vi "程序设置-新建程序.vi"(0 "Program NO.":string) -> (14 "Cancelled?":bool caption="取消？")   [LabVIEW 2017]
doc: "该模板用于创建能够进行事件处理的对话框。"
panel:
  in  "Sequence":bool
  in  "Explanation":string
  in  "Symbol":string
  in  "Index":i32
  out "程序注释 2":string
  out "是否保存":bool
  out "错误输出":errorcluster caption="错误输入"
  in  "程序列表":i32(ring)
  in  "程序注释":string
  in  "Cancel":bool caption="取消"
  in  "Create":bool caption="确定"
  # "新建程序"
  # "程序列表："
  # "程序号  ："
  # "程序注释："
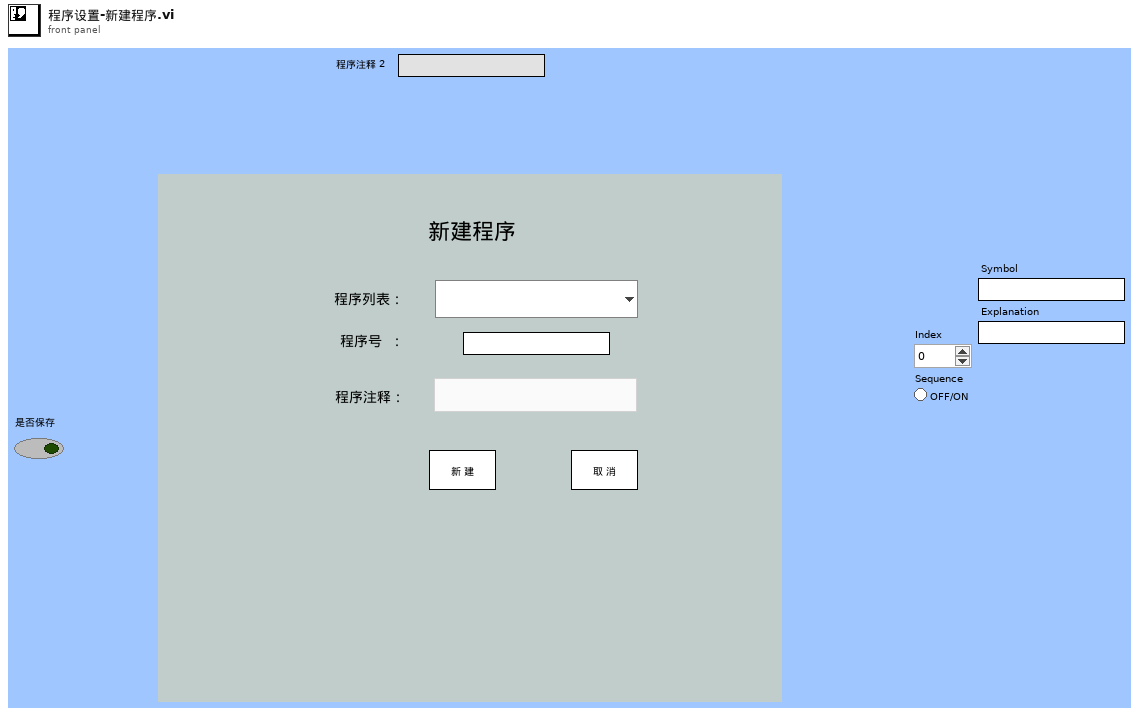
[diagram p1: front panel]
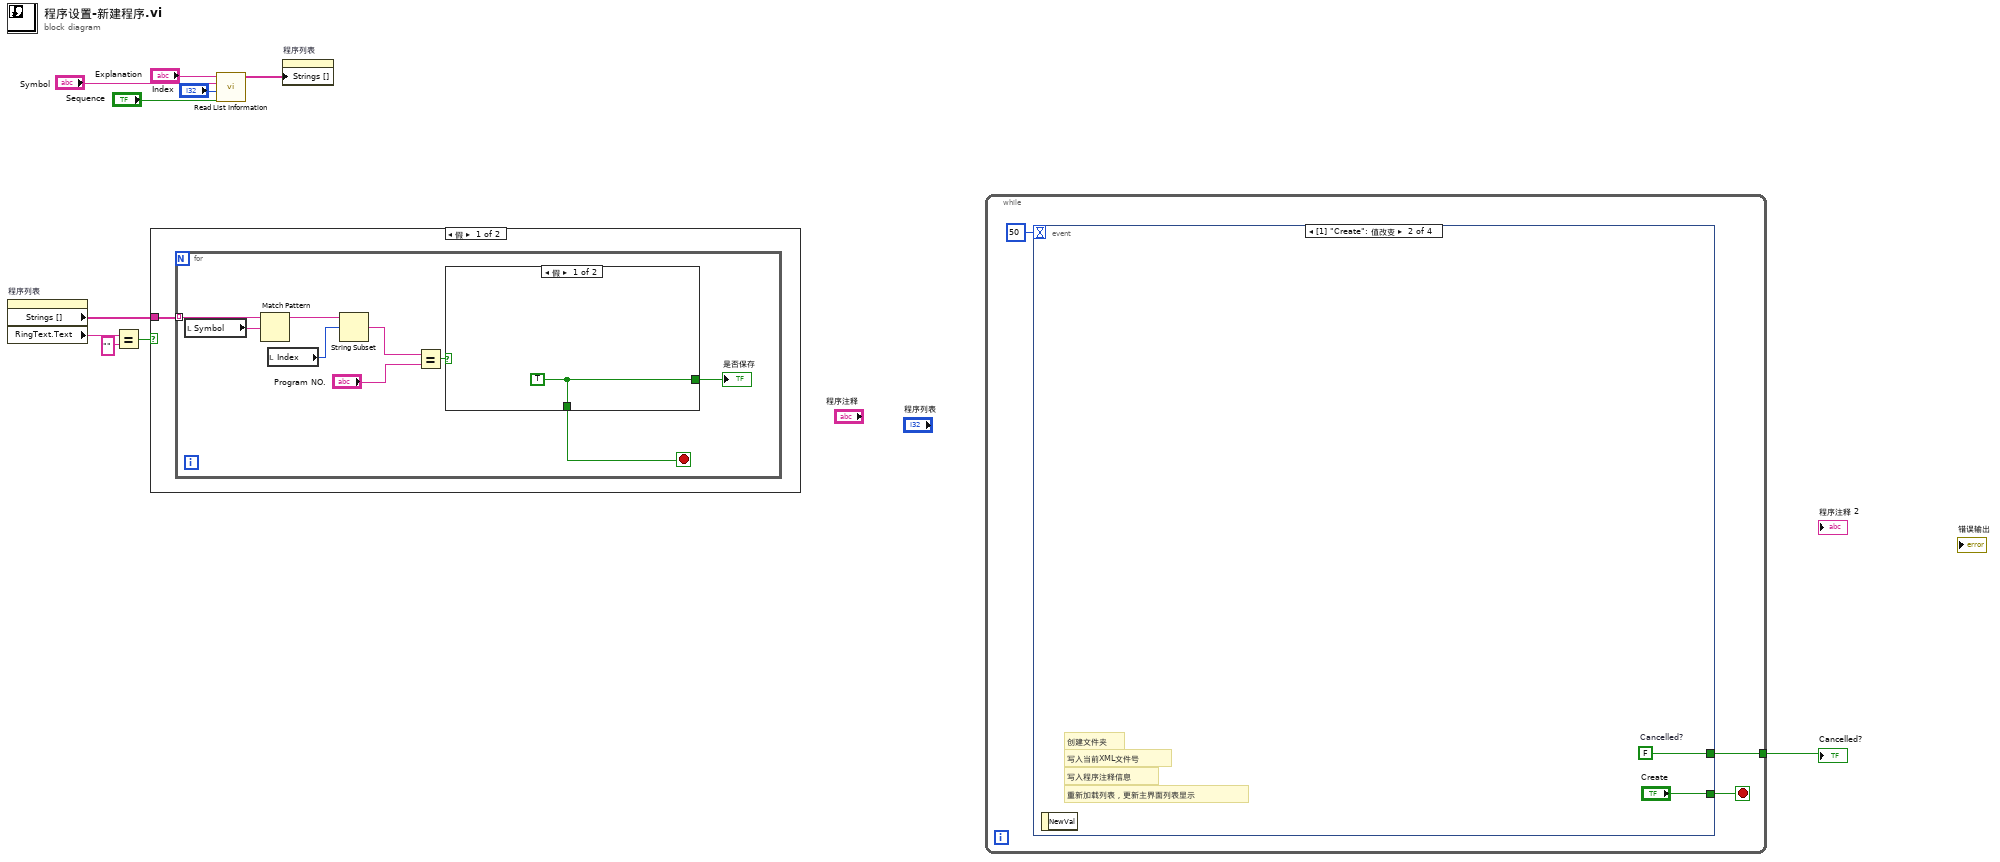
[diagram p0: block diagram]
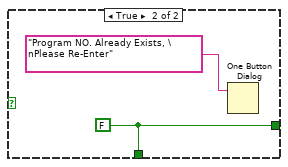
[diagram p2: hidden frame]
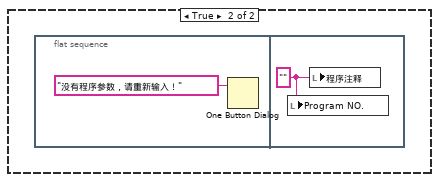
[diagram p3: hidden frame]
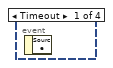
[diagram p4: hidden frame]
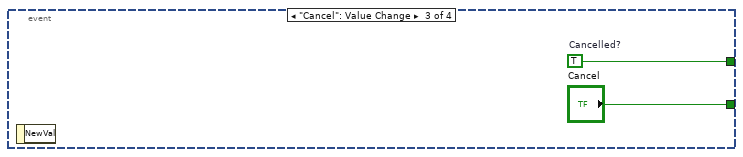
[diagram p5: hidden frame]
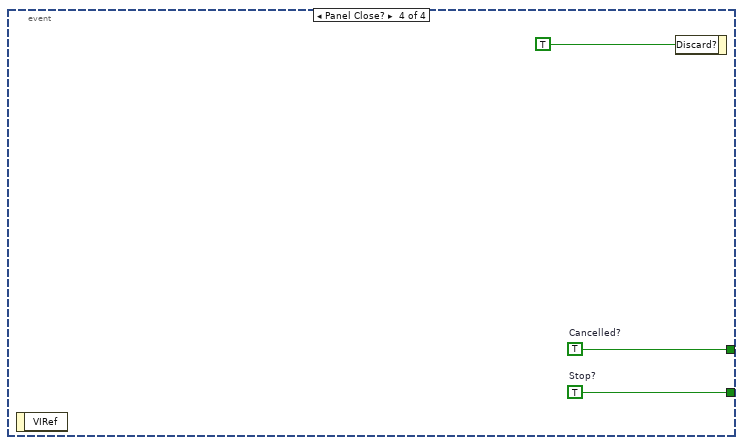
[diagram p6: hidden frame]
diagram:
  n1 = property on="程序列表" class="Ring (严格)"() -> ("Strings []"=w6:string[], "RingText.Text"=w7:string)  [unwired: 2 in, 2 out]
  n2 = Equal?(x=w7, y="") -> (x = y?=w9:bool)
  n3 = case shown="假" w9 {
    tunnel: w6 -> [w11 _]
    frame False {
      n4 = for {
        tunnel: w11 -> [w17] mode=indexing
        stop <- w20 stop-if-true
        n5 = local read "Symbol"() -> (w16:string)
        n6 = Match Pattern(string=w17, regular expression=w16) -> (before substring=w15:string)  [unwired: 1 in, 3 out]
        n7 = local read "Index"() -> (w14:i32)
        n8 = String Subset(string=w15, offset (0)=w14) -> (substring=w13:string)  [unwired: 1 in]
        n9 = Equal?(x=w13, y="Program NO.") -> (x = y?=w18:bool)
        n10 = case shown="假" w18 {
          tunnel: [w21 w23] -> w20
          tunnel: [w21 w23] -> w19
          frame False {
            w21 = TRUE ("程序是否存在")
          }
          frame True {
            w23 = FALSE ("程序是否存在")
            n11 = One Button Dialog(message="Program NO. Already Exists, \nPlease Re-Enter" ("消息")) -> ()  [unwired: 1 in, 1 out]
          }
        }
        "是否保存" <- w19
      }
    }
    frame True {
      n12 = flat-sequence {
        frame #0 {
          n13 = One Button Dialog(message="没有程序参数，请重新输入！" ("消息")) -> ()  [unwired: 1 in, 1 out]
        }
        frame #1 {
          w25 = "" ("程序注释")
          n14 = local write "Program NO."(w25) -> ()
          n15 = local write "程序注释"(w25) -> ()
        }
      }
    }
  }
  n16 = call "Read List Information.vi"("Sequence"="Sequence", "Index"="Index", "Symbol"="Symbol", "Explanation"="Explanation") -> ("Program+NO.+Symbol+Explanation"=w5:string[])  [unwired: 6 in, 1 out]
  n17 = property on="程序列表" class="Ring (严格)"("Strings []"=w5) -> ()  [unwired: 2 in, 2 out]
  n18 = while {
    tunnel: [w27] -> w10
    stop <- w28 stop-if-true
    n19 = event shown="[1] \"Create\": 值改变" {
      selector: _ -> [_ _ _ _]
      dyn-events: _ -> [_ _ _ _]
      timeout: 50 -> [_ _ _ _]
      tunnel: [_ "Create" "Cancel" w34] -> w28
      tunnel: [_ w30 w32 w33] -> w27
      event Timeout {
        n20 = event-data() -> ()  [unwired: 1 in, 1 out]
      }
      event "Create": Value Change {
        w30 = FALSE  # Cancelled?
        # "写入程序注释信息"
        # "重新加载列表，更新主界面列表显示"
        # "写入当前XML文件号"
        # "创建文件夹"
        n21 = event-data() -> ()  [unwired: 1 in, 1 out]
      }
      event "Cancel": Value Change {
        w32 = TRUE  # Cancelled?
        n22 = event-data() -> ()  [unwired: 1 in, 1 out]
      }
      event Panel Close? {
        w33 = TRUE  # Cancelled?
        w34 = TRUE  # Stop?
        n23 = event-data() -> ()  [unwired: 1 in, 1 out]
        n24 = event-data("Discard?"=TRUE) -> ()  [unwired: 1 in, 1 out]
      }
    }
  }
  "Cancelled?" <- w10
